vi "Check_for_Enqueuer.vi"(8 "error in (no error)":errorcluster, 11 "VI ref":refnum<vi>) -> (0 "error out":errorcluster, 2 "Has Enqueuer?":bool, 3 "VI ref out":refnum<vi>)   [LabVIEW 2015]
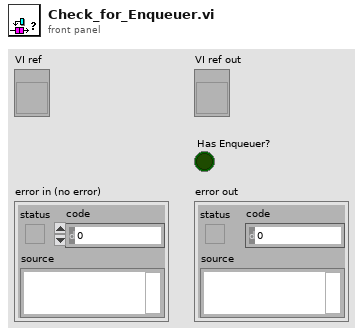
[diagram p1: front panel]
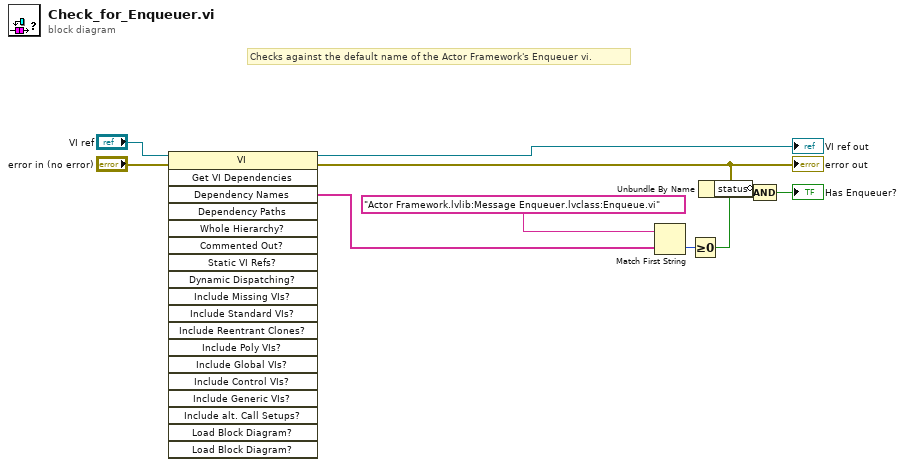
[diagram p0: block diagram]
diagram:
  # "Checks against the default name of the Actor Framework's Enqueuer vi."
  n1 = invoke class="VI" method="Get VI Dependencies"(reference="VI ref", error in="error in (no error)") -> (reference out=→"VI ref out":refnum<vi>, error out=w6:errorcluster, "Dependency Names"=w7:string[])  [unwired: 17 in, 16 out]
  "error out" <- w6
  n2 = Match First String(2:w7, 3:"Actor Framework.lvlib:Message Enqueuer.lvclass:Enqueue.vi") -> (0:w9:i32)  [unwired: 1 out]
  n3 = Greater Or Equal To 0?(x=w9) -> (x >= 0?=w5:bool)
  n4 = Unbundle By Name(w6) -> ("status"=w1:bool)
  n5 = Compound Arithmetic op=AND(invert w1, w5) -> (→"Has Enqueuer?":bool)
